vi "Init Actor.vi"() -> (3 "TEMPLATE Actor out":refnum<class "{{Name}}Actor.lvclass">)   [LabVIEW 2020, in "_Template.lvlib" / "Templates.lvlib" / "{{Name}}Actor.lvlib" / "{{Name}}Actor.lvclass"]
uses:
  {{Name}}Actor.lvclass
  {{Name}}Actor.lvclass/{{Name}}Actor.ctl
panel:
  # "Optionally add controls to the front panel and wire to connector pane terminal postions 10, 9, 6, and/or 4 (the two left middle and two bottom middle terminals for the 4x2x2x4 conn pane)."
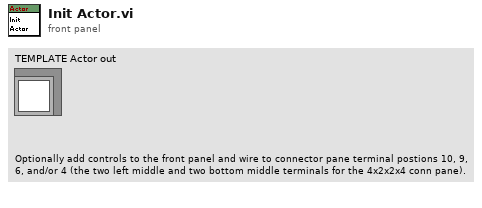
[diagram p1: front panel]
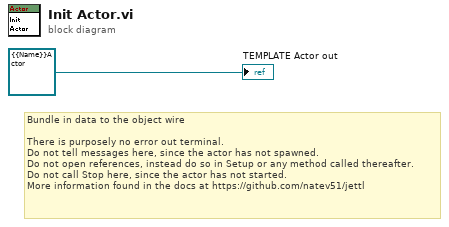
[diagram p0: block diagram]
diagram:
  # "Bundle in data to the object wire\n\nThere is purposely no error out terminal.\nDo not tell messages here, since the actor has not spawned.\nDo not open references, instead do so in Setup or any method called thereafter.\nDo not call Stop here, since the actor has not started.\nMore information found in the docs at https://github.com/natev51/jettl"
  "TEMPLATE Actor out" <- refnum<class "{{Name}}Actor.lvclass"> refnum ("Object")
